vi "ConvertStringToFloat_Array-2D.vi"(11 "params":string[][](array[string])) -> (3 "Array":dbl[][](array[numeric]))   [LabVIEW 2014, in "hse-misc.lvlib"]
doc: "converts array of string values to floating point values\n\n____\nHAMPEL SOFTWARE ENGINEERING v0.11.0 (2018-08-07 00:05)"
uses:
  hse-misc.lvlib
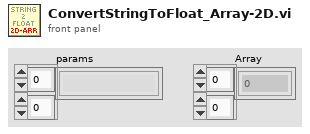
[diagram p1: front panel]
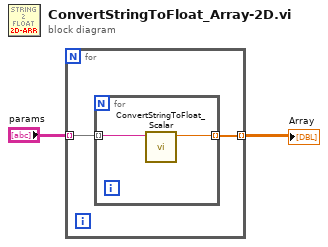
[diagram p0: block diagram]
diagram:
  n1 = for {
    tunnel: "params" -> [w4] mode=indexing
    tunnel: [w3] -> w1 mode=indexing
    n2 = for {
      tunnel: w4 -> [w6] mode=indexing
      tunnel: [w5] -> w3 mode=indexing
      n3 = call "ConvertStringToFloat_Scalar.vi"("String"=w6) -> ("Float"=w5:dbl)  [unwired: 10 in]
    }
  }
  "Array" <- w1
